vi "Initialize Attributes Core.vi"(8 "error in (no error)":errorcluster, 10 "Attribute Data":variant, 11 "BNT_ULx-MCSV-TC in":refnum<class "BNT_ULx-MCSV-TC.lvclass">) -> (0 "error out":errorcluster, 2 "MandatoryParameters":cluster{"Parameter":string, "found?":bool}[](array[cluster]), 3 "BNT_ULx-MCSV-TC out":refnum<class "BNT_ULx-MCSV-TC.lvclass">)   [LabVIEW 2020, in "BNT_ULx.lvlib" / "BNT_ULx-MCSV-TC.lvclass"]
doc: "Initialize object attribute.\n\nUnique resources should be allocated elsewhere!"
uses:
  BNT_ULx-MCSV-TC.lvclass
  BNT_ULx-MCSV-TC.lvclass/BNT_ULx-MCSV-TC.ctl
  BNT_ULx-MCSV/BNT_ULx-MCSV.lvclass
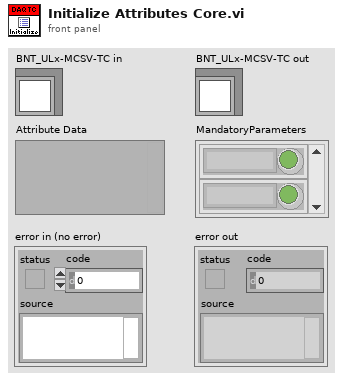
[diagram p1: front panel]
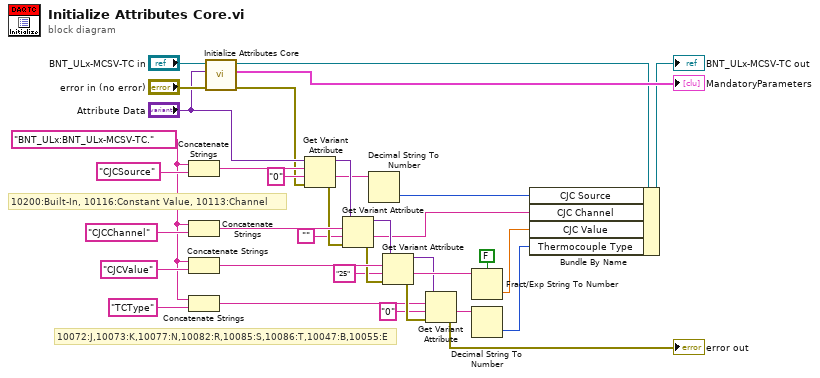
[diagram p0: block diagram]
diagram:
  w15 = "BNT_ULx:BNT_ULx-MCSV-TC."
  # "10072:J,10073:K,10077:N,10082:R,10085:S,10086:T,10047:B,10055:E"
  # "10200:Built-In, 10116:Constant Value, 10113:Channel"
  n1 = Concatenate Strings(w15, "CJCSource" ("string")) -> (w18:string)
  n2 = Concatenate Strings(w15, "CJCChannel" ("string")) -> (w29:string)
  n3 = Concatenate Strings(w15, "CJCValue" ("string")) -> (w27:string)
  n4 = Concatenate Strings(w15, "TCType" ("string")) -> (w22:string)
  n5 = call-parent "Initialize Attributes Core.vi"("error in (no error)"="error in (no error)", "Attribute Data"="Attribute Data", "BNT_ULx-MCSV in"="BNT_ULx-MCSV-TC in") -> ("error out"=w2:errorcluster, "MandatoryParameters"=→"MandatoryParameters":cluster{"Parameter":string, "found?":bool}[], "BNT_ULx-MCSV out"=w13:refnum<class "BNT_ULx-MCSV-TC.lvclass">)  [unwired: 6 in]
  n6 = Get Variant Attribute(Variant="Attribute Data", name=w18, default value (empty Variant)="0", error in=w2) -> (duplicate Variant=w17:variant, value=w11:string, error out=w16:errorcluster)  [unwired: 1 out]
  n7 = Get Variant Attribute(Variant=w17, name=w29, default value (empty Variant)="", error in=w16) -> (duplicate Variant=w28:variant, value=w7:string, error out=w26:errorcluster)  [unwired: 1 out]
  n8 = Decimal String To Number(string=w11) -> (number=w9:i32)  [unwired: 2 in, 1 out]
  n9 = Get Variant Attribute(Variant=w28, name=w27, default value (empty Variant)="25", error in=w26) -> (duplicate Variant=w23:variant, value=w25:string, error out=w24:errorcluster)  [unwired: 1 out]
  n10 = Get Variant Attribute(Variant=w23, name=w22, default value (empty Variant)="0", error in=w24) -> (value=w21:string, error out=→"error out":errorcluster)  [unwired: 2 out]
  n11 = Fract/Exp String To Number(use system decimal point (T)=FALSE, string=w25) -> (number=w5:dbl)  [unwired: 2 in, 1 out]
  n12 = Decimal String To Number(string=w21) -> (number=w3:i32)  [unwired: 2 in, 1 out]
  n13 = Bundle By Name(cluster=w13, "CJC Source"=w9, "CJC Channel"=w7, "CJC Value"=w5, "Thermocouple Type"=w3) -> (→"BNT_ULx-MCSV-TC out":refnum<class "BNT_ULx-MCSV-TC.lvclass">)
